vi "Template RF Test Set Parameters.vi"(8 "error in (no error)":errorcluster, 10 "Parameters":T1, 11 "Template Tx Test in":refnum<class "Template RF Test.lvclass">) -> (0 "error out":errorcluster, 3 "Template Tx Test out":refnum<class "Template RF Test.lvclass">)   [LabVIEW 2015, in "niDTS Template.lvlib" / "Template RF Test.lvclass"]
uses:
  Template RF Test.lvclass
  Includes/Template RF Test INC Parameters.ctl
  Template RF Test.lvclass/Template RF Test.ctl
  niDTS Template.lvlib
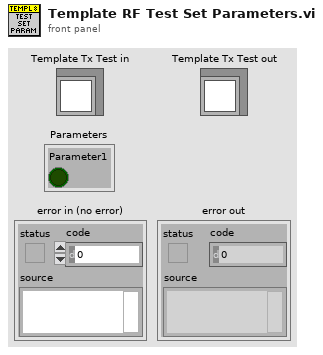
[diagram p1: front panel]
types:
  T1 = typedef "niDTS Template.lvlib/Template RF Test INC Parameters.ctl" = cluster{"Parameter1":bool}
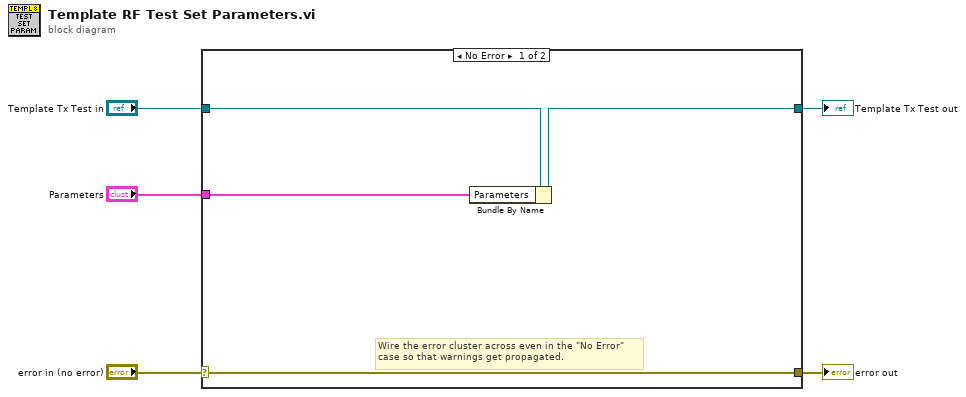
[diagram p0: block diagram]
diagram:
  n1 = case shown="No Error" "error in (no error)" {
    selector: "error in (no error)" -> [w9 w11]
    tunnel: [w9 w11] -> w4
    tunnel: [w7 w10] -> w2
    tunnel: "Template Tx Test in" -> [w8 w10]
    tunnel: "Parameters" -> [w6 _]
    frame No Error {
      # "Wire the error cluster across even in the \"No Error\"\ncase so that warnings get propagated."
      n2 = Bundle By Name(cluster=w8, "Parameters"=w6) -> (w7:refnum<class "Template RF Test.lvclass">)
    }
    frame Error {
    }
  }
  "error out" <- w4
  "Template Tx Test out" <- w2
